vi "IRrangement données brut_SD.vi"(1 "Nombre d'acquisition":i32, 2 "Brut camera":u32[][](graph) caption="Data Values") -> (0 "Data THz1000Hz":u16[](graph) caption="Data Values")   [LabVIEW 2015]
panel:
  in  "y":i32=2
  # "Permet de mettre bout à bout les données qui sortent du Vi ReadFFLoop.vi\nDe type ABAB...\nOn commence le traitement à la deuxième ligne car on coupe la première acquisition qui est bruiteuse (photons accumulés entre deux acquisitions)"
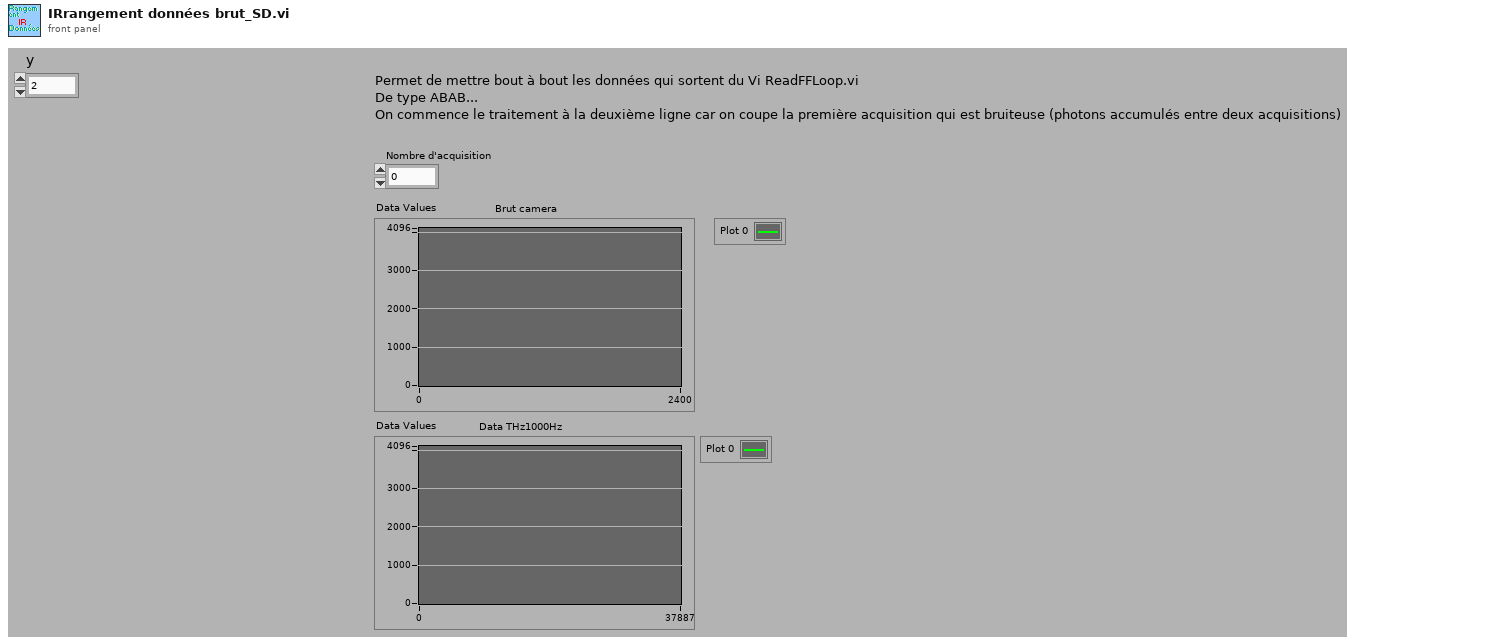
[diagram p1: front panel]
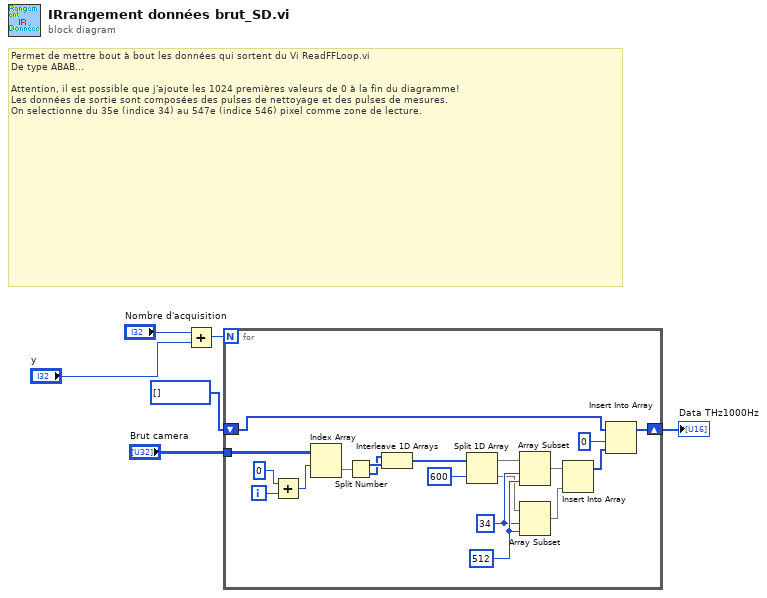
[diagram p0: block diagram]
diagram:
  # "Permet de mettre bout à bout les données qui sortent du Vi ReadFFLoop.vi\nDe type ABAB...\n\nAttention, il est possible que j'ajoute les 1024 premières valeurs de 0 à la fin du diagramme!\nLes données de sortie sont composées des pulses de nettoyage et des pulses de mesures.\nOn selectionne du 35e (indice 34) au 547e (indice 546) pixel comme zone de lecture."
  n1 = Add(x="Nombre d'acquisition", y="y") -> (x+y=w3:i32)
  n2 = for {
    N: w3 -> [_]
    tunnel: "Brut camera" -> [w16]
    shift-right: [w8] -> w2
    shift-left: u16[] [] -> [w9]
    i -> [w17]
    w22 = 34 ("indice")
    w23 = 512 ("longueur")
    n3 = Add(x=0 ("y"), y=w17) -> (x+y=w15:i32)
    n4 = Index Array(array=w16, index (row)=w15) -> (element=w14:u32[])  [unwired: 1 in]
    n5 = Split Number(x=w14) -> (hi(x)=w13:u16[], lo(x)=w12:u16[])
    n6 = Interleave 1D Arrays(w12, w13) -> (w25:u16[])
    n7 = Split 1D Array(array=w25, index=600 ("indice")) -> (first subarray=w20:u16[], second subarray=w19:u16[])
    n8 = Array Subset(array=w20, index=w22, length=w23) -> (w11:u16[])
    n9 = Array Subset(array=w19, index=w22, length=w23) -> (w10:u16[])
    n10 = Insert Into Array(array=w11, new element=w10) -> (w21:u16[])  [unwired: 1 in]
    n11 = Insert Into Array(array=w9, index=0 ("indice"), new element=w21) -> (w8:u16[])
  }
  "Data THz1000Hz" <- w2
